vi "libssh2_session_supported_algs.vi"(8 "error in (no error)":errorcluster, 10 "method_type":T1, 11 "session":T2) -> (0 "error out":errorcluster, 2 "algs":string[](array[string]))   [LabVIEW 2013, in "libssh2.lvlib"]
doc: "Get the supported algorithms for a method type.\n\nFor a list of supported compression algorithms, <B>libssh2_session_flag</B> must be called with LIBSSH2_FLAG_COMPRESS=1. Otherwise, \"none\" will be returned.\n\nIf successful, returns an array with supported algorithms as defined in RFC 4253."
uses:
  libssh2.lvlib
  Session Refnum.ctl
  libssh2_method_type.ctl
  Not A Session.vi
  <vilib>/Utility/error.llb/Error Cluster From Error Code.vi
  Global Settings.vi
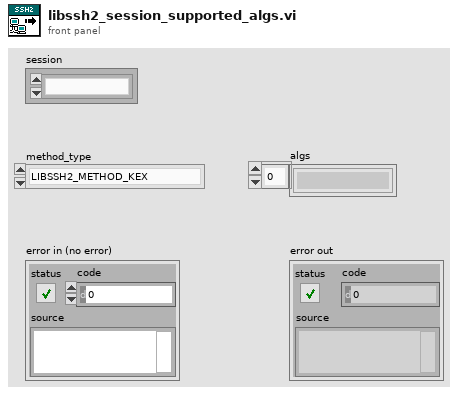
[diagram p1: front panel]
types:
  T1 = typedef "libssh2.lvlib/libssh2_method_type.ctl" = enum16{"LIBSSH2_METHOD_KEX", "LIBSSH2_METHOD_HOSTKEY", "LIBSSH2_METHOD_CRYPT_CS", "LIBSSH2_METHOD_CRYPT_SC", "LIBSSH2_METHOD_MAC_CS", "LIBSSH2_METHOD_MAC_SC", "LIBSSH2_METHOD_COMP_CS", "LIBSSH2_METHOD_COMP_SC", "LIBSSH2_METHOD_LANG_CS", "LIBSSH2_METHOD_LANG_SC", "LIBSSH2_METHOD_SIGN_ALGO"}
  T2 = typedef "libssh2.lvlib/Session Refnum.ctl" = refnum<k1>
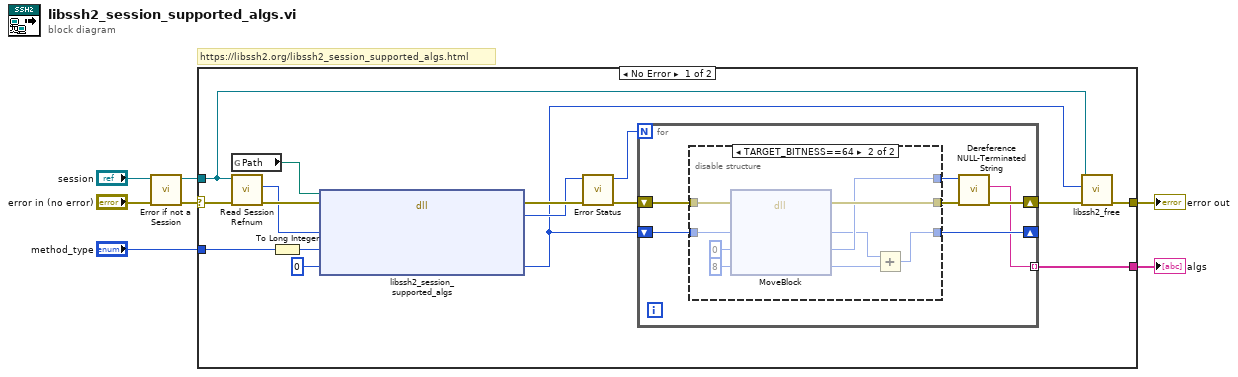
[diagram p0: block diagram]
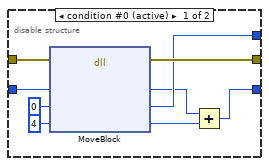
[diagram p2: hidden frame]
diagram:
  # "https://libssh2.org/libssh2_session_supported_algs.html"
  n1 = call "Error if not a Session.vi"("error in (no error)"="error in (no error)", "session"="session") -> ("error out"=w5:errorcluster, "session out"=w3:T2)  [unwired: 8 in]
  n2 = case shown="No Error" w5 {
    selector: w5 -> [w22 w49]
    tunnel: [w12 w49] -> w7
    tunnel: w3 -> [w11 _]
    tunnel: "method_type" -> [w18 _]
    tunnel: [w9 _] -> w1
    frame No Error {
      n3 = global read "Global Settings.vi" "Path"() -> (w19:path)
      n4 = call "Read Session Refnum.vi"("error in (no error)"=w22, "session"=w11) -> ("error out"=w21:errorcluster, "LIBSSH2_SESSION*"=w20:u64)  [unwired: 5 in, 3 out]
      n5 = To Long Integer(number=w18) -> (32bit integer=w17:i32)
      n6 = dll-call lib="?" fn="libssh2_session_supported_algs"(path in=w19, error in=w21, "session"=w20, "method_type"=w17, "algs"=u64 0) -> (error out=w23:errorcluster, "return value"=w16:i32, "algs"=w8:u64)  [unwired: 3 in, 1 out]
      n7 = call "Error Status.vi"("error in (no error)"=w23, "return value"=w16) -> ("error out"=w14:errorcluster, "return value out"=w10:i32)  [unwired: 8 in]
      n8 = for {
        N: w10 -> [_]
        shift-right: [w27] -> w13
        shift-left: w14 -> [w30]
        shift-right: [w25] -> _
        shift-left: w8 -> [w26]
        tunnel: [w24] -> w9 mode=indexing
        n9 = disable-structure shown="TARGET_BITNESS==64" {
          disable-tunnel: w30 -> [w39 w48]
          disable-tunnel: [w38 w47] -> w29
          disable-tunnel: [w35 w44] -> w28
          disable-tunnel: w26 -> [w34 w43]
          disable-tunnel: [w32 w41] -> w25
          frame condition #0 (active) {
            n10 = dll-call lib="LabVIEW" fn="MoveBlock"(error in=w39, "ps"=w34, u64 0, "size"=i64 4) -> (error out=w38:errorcluster, "ps"=w33:u64, w35:u64, "size"=w31:i64)  [unwired: 3 in, 1 out]
            n11 = Add(x=w33, y=w31) -> (x+y=w32:u64)
          }
          frame condition #1 {
            n12 = dll-call lib="LabVIEW" fn="MoveBlock"(error in=w48, "ps"=w43, u64 0, "size"=i64 8) -> (error out=w47:errorcluster, "ps"=w42:u64, w44:u64, "size"=w40:i64)  [unwired: 3 in, 1 out]
            n13 = Add(x=w42, y=w40) -> (x+y=w41:u64)
          }
        }
        n14 = call "Dereference NULL-Terminated String.vi"("error in (no error)"=w29, "char*"=w28) -> ("error out"=w27:errorcluster, "string"=w24:string)  [unwired: 8 in]
      }
      n15 = call "libssh2_free.vi"("error in (no error)"=w13, "ptr"=w8, "session"=w11) -> ("error out"=w12:errorcluster)  [unwired: 8 in]
    }
    frame Error {
    }
  }
  "error out" <- w7
  "algs" <- w1
